vi "PathPlanner_Segment_FindConstraintZone.vi"(9 "T":dbl, 10 "Zones":T1[](array[typedef]), 11 "Segment":T3 {"SegmentPoints"."HolonomicRotation"."SIN" format="%13.4f"; "SegmentPoints"."HolonomicRotation"."COS" format="%13.4f"; "SegmentPoints"."HolonomicRotation"."VALUE" format="%13.4f"; "SegmentPoints"."Position"."Y" format="%14.3f"; "SegmentPoints"."Position"."X" format="%14.3f"}) -> (1 "IsPresent":bool, 3 "Returned Zones":T1[](array[typedef]))   [LabVIEW 2019, in "PathPlanner24.lvlib"]
doc: "/**\n * Create a new path constraints object\n *\n * @param maxVelocityMps Max linear velocity (M/S)\n * @param maxAccelerationMpsSq Max linear acceleration (M/S^2)\n * @param maxAngularVelocityRps Max angular velocity (Rad/S)\n * @param maxAngularAccelerationRpsSq Max angular acceleration (Rad/S^2)\n */"
uses:
  TypeDef/PathPlannerSegment.ctl
  TypeDef/PathPlannerPoint.ctl
  <vilib>/Rock Robotics/WPI/ThirdParty/JAS_Junk/TrajLib/TypeDef/TRANSLATION2D.ctl
  <vilib>/Rock Robotics/WPI/ThirdParty/JAS_Junk/TrajLib/TypeDef/ROTATION2D.ctl
  TypeDef/PathPlannerConstraints.ctl
  PathPlanner24.lvlib
  TypeDef/PathPlannerConstraintsZone.ctl
  <vilib>/Rock Robotics/WPI/ThirdParty/JAS_Junk/TrajLib/Trajectory_Library.lvlib
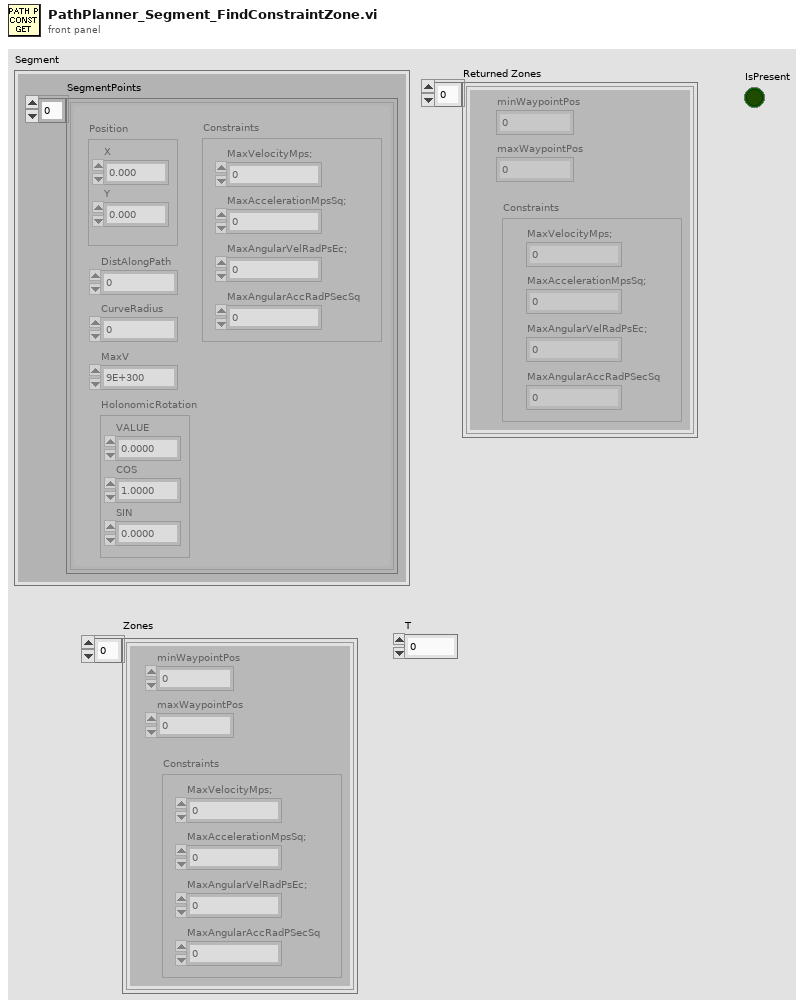
[diagram p1: front panel]
types:
  T1 = typedef "PathPlanner24.lvlib/PathPlannerConstraintsZone.ctl" = cluster{"minWaypointPos":dbl, "maxWaypointPos":dbl, "Constraints":T2}
  T2 = typedef "PathPlanner24.lvlib/PathPlannerConstraints.ctl" = cluster{"MaxVelocityMps;":dbl, "MaxAccelerationMpsSq;":dbl, "MaxAngularVelRadPsEc;":dbl, "MaxAngularAccRadPSecSq":dbl}
  T3 = typedef "PathPlanner24.lvlib/PathPlannerSegment.ctl" = cluster{"SegmentPoints":T4[]}
  T4 = typedef "PathPlanner24.lvlib/PathPlannerPoint.ctl" = cluster{"Position":T5, "HolonomicRotation":T6, "DistAlongPath":dbl, "CurveRadius":dbl, "MaxV":dbl, "Constraints":T2}
  T5 = typedef "Trajectory_Library.lvlib/TRANSLATION2D.ctl" = cluster{"X":dbl, "Y":dbl}
  T6 = typedef "Trajectory_Library.lvlib/ROTATION2D.ctl" = cluster{"VALUE":dbl, "COS":dbl, "SIN":dbl}
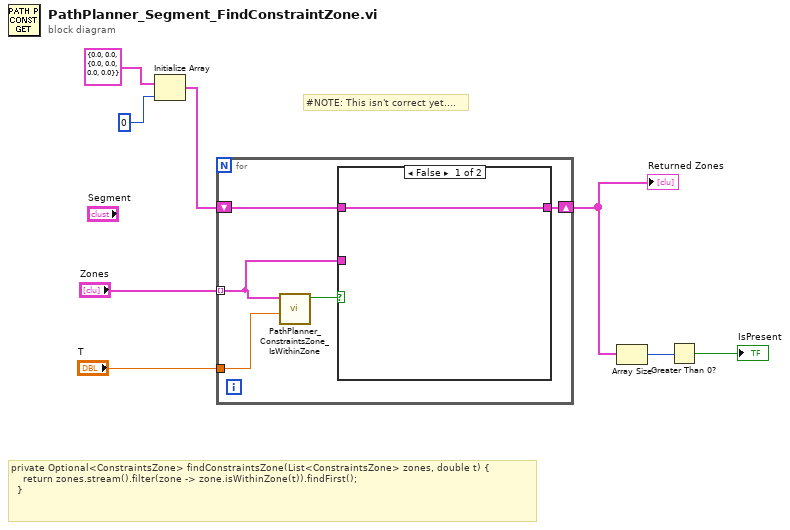
[diagram p0: block diagram]
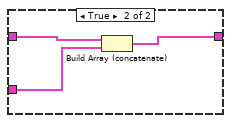
[diagram p2: hidden frame]
diagram:
  # "#NOTE: This isn't correct yet...."
  # "private Optional<ConstraintsZone> findConstraintsZone(List<ConstraintsZone> zones, double t) {\n    return zones.stream().filter(zone -> zone.isWithinZone(t)).findFirst();\n  }"
  n1 = Initialize Array(T1 {"minWaypointPos"=0.0, "maxWaypointPos"=0.0, "Constraints"={"MaxVelocityMps;"=0.0, "MaxAccelerationMpsSq;"=0.0, "MaxAngularVelRadPsEc;"=0.0, "MaxAngularAccRadPSecSq"=0.0}} ("ConstraintsZone"), 0 ("dimension size")) -> (w4:T1[])
  n2 = for {
    tunnel: "T" -> [w13]
    tunnel: "Zones" -> [w11] mode=indexing
    shift-right: [w9] -> w1
    shift-left: w4 -> [w10]
    n3 = call "PathPlanner_ConstraintsZone_IsWithinZone.vi"("T"=w13, "ConstraintsZone"=w11) -> ("WithinZone"=w12:bool)  [unwired: 9 in]
    n4 = case shown="False" w12 {
      tunnel: w11 -> [_ w16]
      tunnel: w10 -> [w14 w17]
      tunnel: [w14 w15] -> w9
      frame False {
      }
      frame True {
        n5 = Build Array (concatenate)(w17, w16) -> (w15:T1[])
      }
    }
  }
  "Returned Zones" <- w1
  n6 = Array Size(array=w1) -> (size(s)=w3:i32)
  n7 = Greater Than 0?(x=w3) -> (x > 0?=→"IsPresent":bool)
